vi "Write Timestamp.vi"(8 "error in (no error)":errorcluster, 9 "Timestamp Value":timestamp, 10 "Hierarchy":string[](array[string]), 11 "Config Manager in":refnum<class "Config Manager.lvclass">) -> (0 "error out":errorcluster, 3 "Config Manager out":refnum<class "Config Manager.lvclass">)   [LabVIEW 2020, in "CDM-Config.lvlib" / "Config Manager.lvclass"]
uses:
  Config Manager.lvclass
  Config Element/Config Element.lvclass
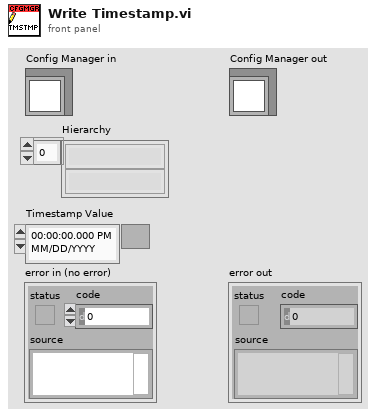
[diagram p1: front panel]
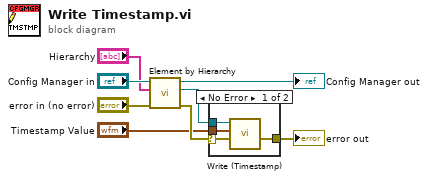
[diagram p0: block diagram]
diagram:
  n1 = call "Element by Hierarchy.vi"("error in (no error)"="error in (no error)", "Hierarchy"="Hierarchy", "Config Manager in"="Config Manager in") -> ("error out"=w4:errorcluster, "Config Element"=w3:refnum<class "Config Element.lvclass">, "Config Manager out"=→"Config Manager out":refnum<class "Config Manager.lvclass">)  [unwired: 6 in]
  n2 = case shown="No Error" w4 {
    selector: w4 -> [w11 w13]
    tunnel: w3 -> [w12 _]
    tunnel: "Timestamp Value" -> [w10 _]
    tunnel: [w9 w13] -> w1
    frame No Error {
      n3 = call "Write (Timestamp).vi"("error in (no error)"=w11, "Timestamp Value"=w10, "Config Element in"=w12) -> ("error out"=w9:errorcluster)  [unwired: 7 in, 1 out]
    }
    frame Error {
    }
  }
  "error out" <- w1
